vi "MKS_PRESSURE (SubVI).vi"(8 "error in (no error)":errorcluster, 11 "Cluster in":T1 caption="Cluster 2" {"parity (0:none)" items=["None", "Odd", "Even", "Mark", "Space"]; "BAUDE RATE" items=["38400"=38400, "19200"=19200, "9600"=9600, "4800"=4800]}) -> (0 "error out":errorcluster, 3 "DBL out":dbl[](array[numeric]))   [LabVIEW 2020]
uses:
  INITIALIZATION.ctl
  <vilib>/Instr/_visa.llb/VISA Configure Serial Port (Instr).vi
  <instrlib>/PV ActiveLine/PV ActiveLine.lvlib
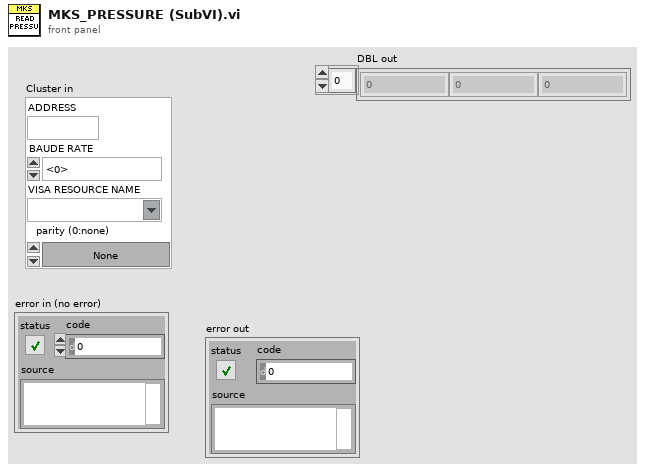
[diagram p1: front panel]
types:
  T1 = typedef "INITIALIZATION.ctl" = cluster{"ADDRESS":string, "BAUDE RATE":u32, "VISA RESOURCE NAME":refnum<visa-resource-name>, "parity (0:none)":u16}
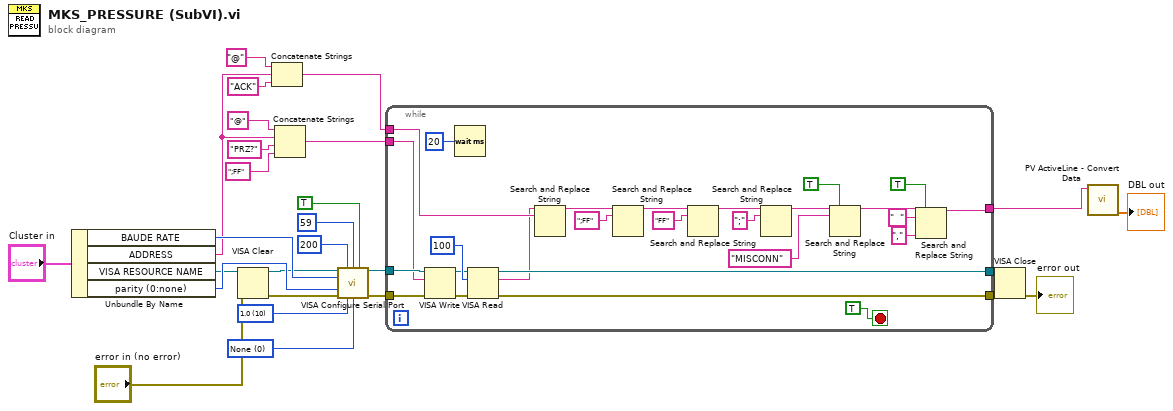
[diagram p0: block diagram]
diagram:
  w17 = u16 0 items=["None", "XON/XOFF", "RTS/CTS", "XON/XOFF & RTS/CTS", "DTR/DSR", "XON/XOFF & DTR/DSR"] ("flow control (0:none)")
  w23 = u16 10 items=["1.0"=10, "1.5"=15, "2.0"=20] ("stop bits (10: 1 bit)")
  n1 = Unbundle By Name("Cluster in") -> ("BAUDE RATE"=w22:u32, "ADDRESS"=w15:string, "VISA RESOURCE NAME"=w5:refnum<visa-resource-name>, "parity (0:none)"=w16:u16)
  n2 = VISA Clear(VISA resource name=w5, error in (no error)="error in (no error)") -> (VISA resource name out=w6:refnum<visa-resource-name>, error out=w4:errorcluster)
  n3 = Concatenate Strings("@" ("search string"), w15, "ACK" ("string")) -> (w7:string)
  n4 = Concatenate Strings("@" ("string"), w15, "PRZ?" ("string"), ";FF" ("string")) -> (w10:string)
  n5 = call-poly "VISA Configure Serial Port"("VISA resource name"=w6, "timeout (10sec)"=u32 200, "termination char\n(0xA = '\\n' = LF)"=u8 59, "Enable Termination\nChar (T)"=TRUE ("Enable Termination\nChar (T)"), "baud rate (9600)"=w22, "parity (0:none)"=w16, "error in (no error)"=w4, "stop bits (10: 1 bit)"=w23, "flow control (0:none)"=w17) -> ("VISA resource name out"=w19:refnum<visa-resource-name>, "error out"=w18:errorcluster)  [unwired: 5 in]
  n6 = while {
    tunnel: w18 -> [w53]
    tunnel: [w51] -> w14
    tunnel: w19 -> [w52]
    tunnel: [w50] -> w27
    tunnel: w10 -> [w33]
    tunnel: w7 -> [w44]
    tunnel: [w31] -> w3
    stop <- TRUE stop-if-true
    n7 = VISA Write(VISA resource name=w52, write buffer=w33, error in (no error)=w53) -> (VISA resource name out=w39:refnum<visa-resource-name>, error out=w38:errorcluster)  [unwired: 1 out]
    n8 = Wait (ms)(milliseconds to wait=u32 20) -> ()  [unwired: 1 out]
    n9 = VISA Read(VISA resource name=w39, byte count=u32 100, error in (no error)=w38) -> (VISA resource name out=w50:refnum<visa-resource-name>, read buffer=w34:string, error out=w51:errorcluster)  [unwired: 1 out]
    n10 = Search and Replace String(input string=w34, search string=w44) -> (result string=w47:string)  [unwired: 6 in, 3 out]
    n11 = Search and Replace String(input string=w47, search string=";FF") -> (result string=w41:string)  [unwired: 6 in, 3 out]
    n12 = Search and Replace String(input string=w41, search string="FF") -> (result string=w40:string)  [unwired: 6 in, 3 out]
    n13 = Search and Replace String(input string=w40, search string=";") -> (result string=w37:string)  [unwired: 6 in, 3 out]
    n14 = Search and Replace String(replace all?=TRUE ("replace all? (F)"), input string=w37, search string="MISCONN") -> (result string=w32:string)  [unwired: 5 in, 3 out]
    n15 = Search and Replace String(replace all?=TRUE ("replace all? (F)"), input string=w32, search string="  ", replace string="," ("replace string (\"\")")) -> (result string=w31:string)  [unwired: 4 in, 3 out]
  }
  n16 = VISA Close(VISA resource name=w27, error in (no error)=w14) -> (error out=→"error out":errorcluster)
  n17 = call <instrlib>:"PV ActiveLine - Convert Data.vi"("String in"=w3) -> ("DBL out"=→"DBL out":dbl[])  [unwired: 7 in, 3 out]
